vi "Timestamp I2C.vi"(0 "timestamp counter value":T2, 1 "reset":bool, 5 "i2c monitor array":T1[](array[typedef]) {"monitor word" format="%.0x"}) -> (4 "user timestamp fifo overflow":bool)   [LabVIEW 2020, in "GettingStarted_Common_148X_FPGA.lvlib"]
uses:
  GettingStarted_Common_148X_FPGA.lvlib
  <instrlib>/FlexRIO/CSI-2/v2/FPGA/Types/Timestamp Counter Value.ctl
  <instrlib>/FlexRIO/API/FPGA/v1/IO/NI148x/i2c monitor.ctl
  <instrlib>/_niInstr/Basic Elements/v1/FPGA/Private/Write U64 FIFO.vi
  <instrlib>/_niInstr/Basic Elements/v1/FPGA/niInstr Basic Elements v1 FPGA.lvlib
  <instrlib>/FlexRIO/CSI-2/v2/FPGA/NI CSI-2 API FPGA v2.lvlib
  <instrlib>/FlexRIO/CSI-2/v2/FPGA/subVIs/Convert User Timestamp to Raw Timestamp.vi
  <instrlib>/FlexRIO/CSI-2/v2/FPGA/Types/Timestamp ID.ctl
  <instrlib>/FlexRIO/API/FPGA/v1/IO/NI148x/FlexRIO 148x FPGA v1.lvlib
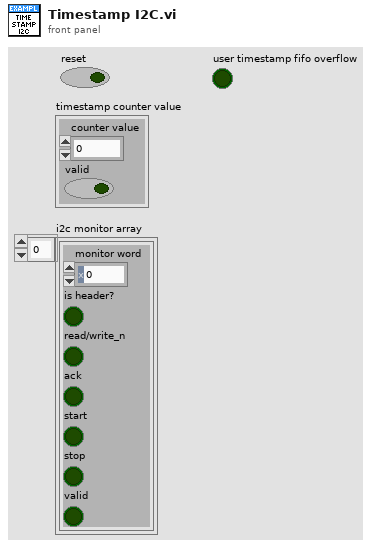
[diagram p1: front panel]
types:
  T1 = typedef "FlexRIO 148x FPGA v1.lvlib/i2c monitor.ctl" = cluster{"monitor word":u8, "is header?":bool, "read/write_n":bool, "ack":bool, "start":bool, "stop":bool, "valid":bool}
  T2 = typedef "NI CSI-2 API FPGA v2.lvlib/Timestamp Counter Value.ctl" = cluster{"counter value":u64, "valid":bool}
  T3 = typedef "NI CSI-2 API FPGA v2.lvlib/Timestamp ID.ctl" = enum8{"SI0 LLP", "SI1 LLP", "SI2 LLP", "SI3 LLP", "SI4 LLP", "SI5 LLP", "SI6 LLP", "SI7 LLP", "SO0 LLP", "SO1 LLP", "SO2 LLP", "SO3 LLP", "SO4 LLP", "SO5 LLP", "SO6 LLP", "SO7 LLP", "Ser0 GPIO Bank", "Ser1 GPIO Bank", "Ser2 GPIO Bank", "Ser3 GPIO Bank", "Ser4 GPIO Bank", "Ser5 GPIO Bank", "Ser6 GPIO Bank", "Ser7 GPIO Bank", "Des0 GPIO Bank", "Des1 GPIO Bank", "Des2 GPIO Bank", "Des3 GPIO Bank", "Des4 GPIO Bank", "Des5 GPIO Bank", "Des6 GPIO Bank", "Des7 GPIO Bank", "User0", "User1", "User2", "User3", "User4", "User5", "User6", "User7", "User8", "User9", "User10", "User11", "User12", "User13", "User14", "User15", "User16", "User17", "User18", "User19", "User20", "User21", "User22", "User23", "User24", "User25", "User26", "User27", "User28", "User29", "User30", "User31"}
  T4 = typedef "NI CSI-2 API FPGA v2.lvlib/User Timestamp.ctl" = cluster{"valid":bool, "user data":fxp<+,58,58>, "id":T3}
  T5 = typedef "NI CSI-2 API FPGA v2.lvlib/Raw Timestamp.ctl" = cluster{"timestamp":u64, "valid":bool}
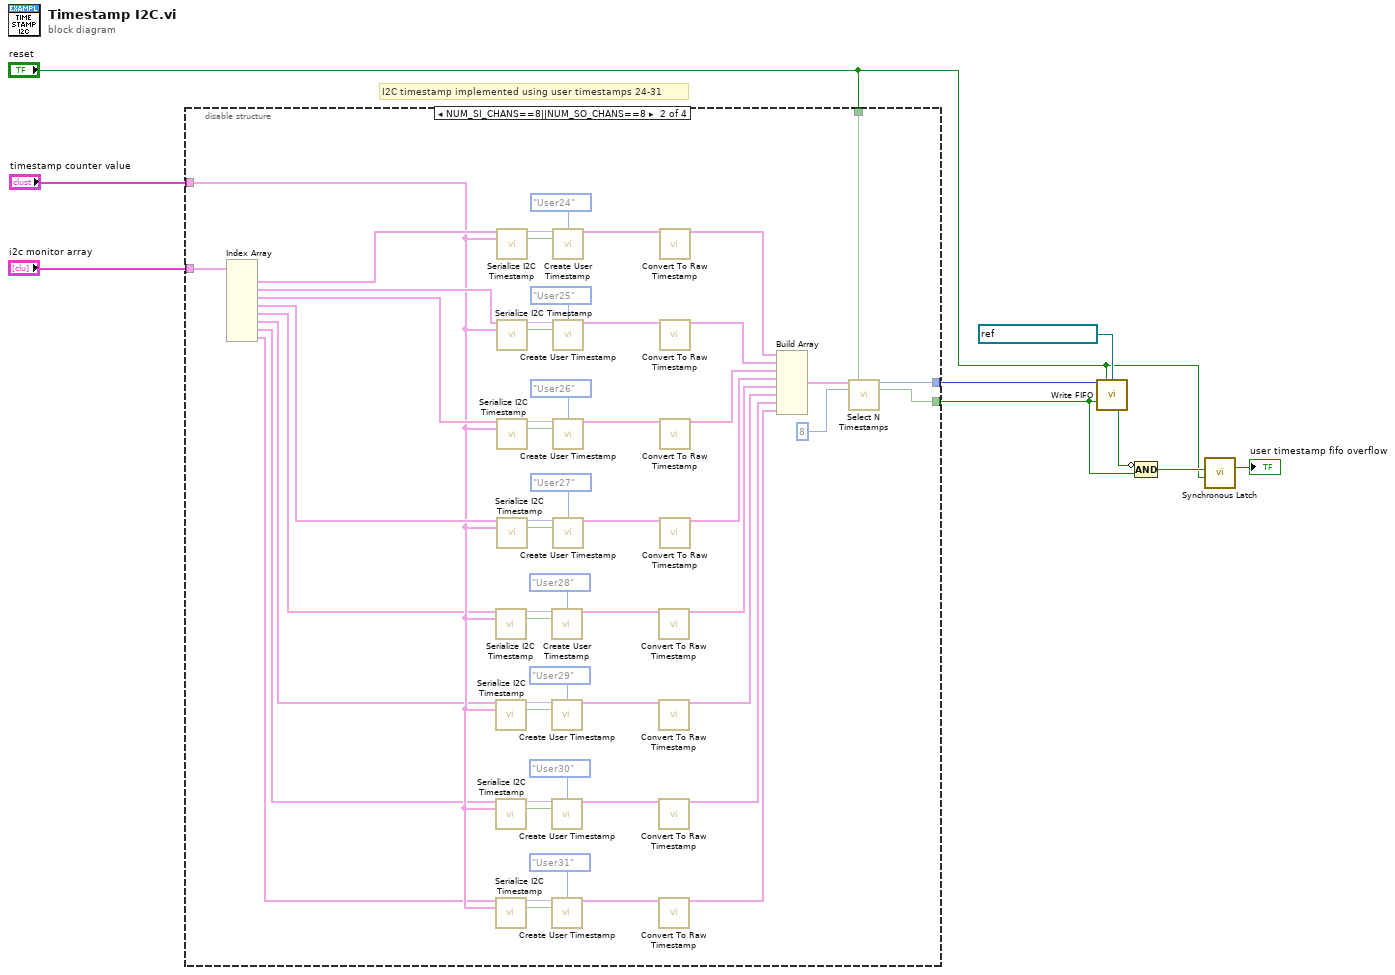
[diagram p0: block diagram]
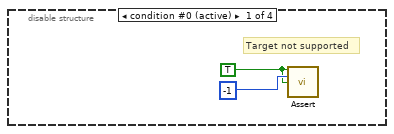
[diagram p2: hidden frame]
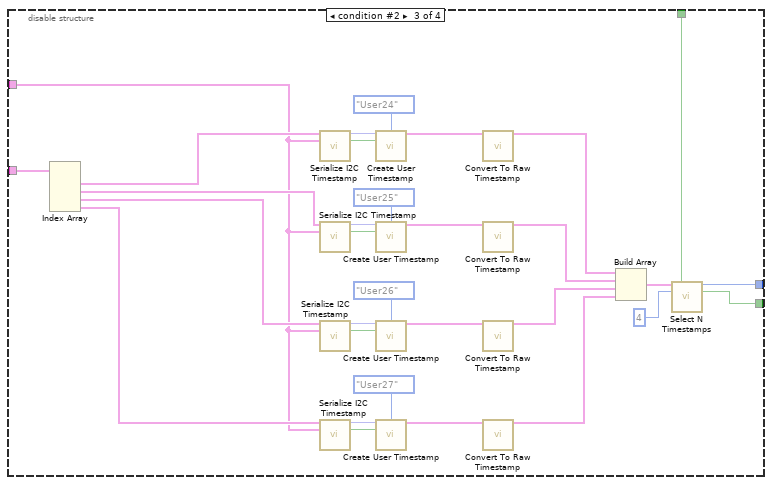
[diagram p3: hidden frame]
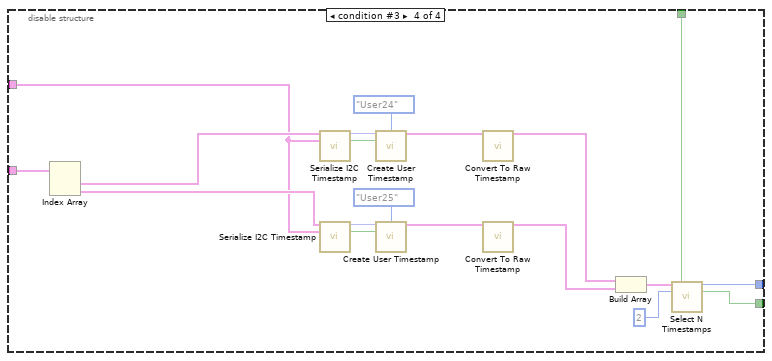
[diagram p4: hidden frame]
diagram:
  # "I2C timestamp implemented using user timestamps 24-31"
  n1 = disable-structure shown="NUM_SI_CHANS==8||NUM_SO_CHANS==8" {
    disable-tunnel: "i2c monitor array" -> [_ w42 w73 w104]
    disable-tunnel: "timestamp counter value" -> [_ w25 w72 w103]
    disable-tunnel: [_ w16 w70 w101] -> w3
    disable-tunnel: [_ w15 w69 w100] -> w2
    disable-tunnel: "reset" -> [_ w14 w68 w99]
    frame condition #0 (active) {
      w10 = TRUE ("assert")
      # "Target not supported"
      n2 = call <instrlib>:"Assert.vi"("assert"=w10, "error code"=-1, "enable show error"=w10) -> ()  [unwired: 13 in]
    }
    frame condition #1 {
      n3 = Index Array(array=w42) -> (element #1=w47:T1, element #2=w49:T1, element #3=w50:T1, element #4=w51:T1, element #5=w24:T1, element #6=w23:T1, element #7=w22:T1, element #8=w21:T1)  [unwired: 8 in]
      n4 = call "Serialize I2C Timestamp.vi"("i2c monitor"=w24, "timestamp counter value"=w25) -> ("data"=w39:fxp<+,58,58>, "create timestamp"=w38:bool)  [unwired: 12 in]
      n5 = call "Serialize I2C Timestamp.vi"("i2c monitor"=w23, "timestamp counter value"=w25) -> ("data"=w37:fxp<+,58,58>, "create timestamp"=w36:bool)  [unwired: 12 in]
      n6 = call "Serialize I2C Timestamp.vi"("i2c monitor"=w22, "timestamp counter value"=w25) -> ("data"=w35:fxp<+,58,58>, "create timestamp"=w34:bool)  [unwired: 12 in]
      n7 = call "Serialize I2C Timestamp.vi"("i2c monitor"=w21, "timestamp counter value"=w25) -> ("data"=w33:fxp<+,58,58>, "create timestamp"=w32:bool)  [unwired: 12 in]
      n8 = call "Serialize I2C Timestamp.vi"("i2c monitor"=w47, "timestamp counter value"=w25) -> ("data"=w45:fxp<+,58,58>, "create timestamp"=w46:bool)  [unwired: 12 in]
      n9 = call "Serialize I2C Timestamp.vi"("i2c monitor"=w49, "timestamp counter value"=w25) -> ("data"=w52:fxp<+,58,58>, "create timestamp"=w53:bool)  [unwired: 12 in]
      n10 = call "Serialize I2C Timestamp.vi"("i2c monitor"=w50, "timestamp counter value"=w25) -> ("data"=w54:fxp<+,58,58>, "create timestamp"=w55:bool)  [unwired: 12 in]
      n11 = call "Serialize I2C Timestamp.vi"("i2c monitor"=w51, "timestamp counter value"=w25) -> ("data"=w56:fxp<+,58,58>, "create timestamp"=w57:bool)  [unwired: 12 in]
      n12 = call <instrlib>:"Create User Timestamp.vi"("user data"=w39, "timestamp id"=Timestamp_ID."User28" ("id"), "create timestamp"=w38) -> ("user timestamp"=w41:T4)  [unwired: 12 in]
      n13 = call <instrlib>:"Create User Timestamp.vi"("user data"=w37, "timestamp id"=Timestamp_ID."User29" ("id"), "create timestamp"=w36) -> ("user timestamp"=w29:T4)  [unwired: 12 in]
      n14 = call <instrlib>:"Create User Timestamp.vi"("user data"=w35, "timestamp id"=Timestamp_ID."User30" ("id"), "create timestamp"=w34) -> ("user timestamp"=w30:T4)  [unwired: 12 in]
      n15 = call <instrlib>:"Create User Timestamp.vi"("user data"=w33, "timestamp id"=Timestamp_ID."User31" ("id"), "create timestamp"=w32) -> ("user timestamp"=w31:T4)  [unwired: 12 in]
      n16 = call <instrlib>:"Create User Timestamp.vi"("user data"=w45, "timestamp id"=Timestamp_ID."User24" ("id"), "create timestamp"=w46) -> ("user timestamp"=w43:T4)  [unwired: 12 in]
      n17 = call <instrlib>:"Create User Timestamp.vi"("user data"=w52, "timestamp id"=Timestamp_ID."User25" ("id"), "create timestamp"=w53) -> ("user timestamp"=w60:T4)  [unwired: 12 in]
      n18 = call <instrlib>:"Create User Timestamp.vi"("user data"=w54, "timestamp id"=Timestamp_ID."User26" ("id"), "create timestamp"=w55) -> ("user timestamp"=w59:T4)  [unwired: 12 in]
      n19 = call <instrlib>:"Create User Timestamp.vi"("user data"=w56, "timestamp id"=Timestamp_ID."User27" ("id"), "create timestamp"=w57) -> ("user timestamp"=w58:T4)  [unwired: 12 in]
      n20 = call-poly <instrlib>:"Convert To Raw Timestamp.vi"("user timestamp"=w41) -> ("raw timestamp"=w20:T5)  [unwired: 14 in]
      n21 = call-poly <instrlib>:"Convert To Raw Timestamp.vi"("user timestamp"=w29) -> ("raw timestamp"=w19:T5)  [unwired: 14 in]
      n22 = call-poly <instrlib>:"Convert To Raw Timestamp.vi"("user timestamp"=w30) -> ("raw timestamp"=w18:T5)  [unwired: 14 in]
      n23 = call-poly <instrlib>:"Convert To Raw Timestamp.vi"("user timestamp"=w31) -> ("raw timestamp"=w17:T5)  [unwired: 14 in]
      n24 = call-poly <instrlib>:"Convert To Raw Timestamp.vi"("user timestamp"=w43) -> ("raw timestamp"=w48:T5)  [unwired: 14 in]
      n25 = call-poly <instrlib>:"Convert To Raw Timestamp.vi"("user timestamp"=w60) -> ("raw timestamp"=w61:T5)  [unwired: 14 in]
      n26 = call-poly <instrlib>:"Convert To Raw Timestamp.vi"("user timestamp"=w59) -> ("raw timestamp"=w62:T5)  [unwired: 14 in]
      n27 = call-poly <instrlib>:"Convert To Raw Timestamp.vi"("user timestamp"=w58) -> ("raw timestamp"=w63:T5)  [unwired: 14 in]
      n28 = Build Array(w48, w61, w62, w63, w20, w19, w18, w17) -> (w13:T5[])
      n29 = call <instrlib>:"Select N Timestamps.vi"("raw timestamps"=w13, "reset"=w14, "number of timestamps"=u8 8) -> ("timestamp"=w16:u64, "output valid"=w15:bool)  [unwired: 11 in]
    }
    frame condition #2 {
      n30 = Index Array(array=w73) -> (element #1=w78:T1, element #2=w80:T1, element #3=w81:T1, element #4=w82:T1)  [unwired: 4 in]
      n31 = call "Serialize I2C Timestamp.vi"("i2c monitor"=w78, "timestamp counter value"=w72) -> ("data"=w76:fxp<+,58,58>, "create timestamp"=w77:bool)  [unwired: 12 in]
      n32 = call "Serialize I2C Timestamp.vi"("i2c monitor"=w80, "timestamp counter value"=w72) -> ("data"=w83:fxp<+,58,58>, "create timestamp"=w84:bool)  [unwired: 12 in]
      n33 = call "Serialize I2C Timestamp.vi"("i2c monitor"=w81, "timestamp counter value"=w72) -> ("data"=w85:fxp<+,58,58>, "create timestamp"=w86:bool)  [unwired: 12 in]
      n34 = call "Serialize I2C Timestamp.vi"("i2c monitor"=w82, "timestamp counter value"=w72) -> ("data"=w87:fxp<+,58,58>, "create timestamp"=w88:bool)  [unwired: 12 in]
      n35 = call <instrlib>:"Create User Timestamp.vi"("user data"=w76, "timestamp id"=Timestamp_ID."User24" ("id"), "create timestamp"=w77) -> ("user timestamp"=w74:T4)  [unwired: 12 in]
      n36 = call <instrlib>:"Create User Timestamp.vi"("user data"=w83, "timestamp id"=Timestamp_ID."User25" ("id"), "create timestamp"=w84) -> ("user timestamp"=w91:T4)  [unwired: 12 in]
      n37 = call <instrlib>:"Create User Timestamp.vi"("user data"=w85, "timestamp id"=Timestamp_ID."User26" ("id"), "create timestamp"=w86) -> ("user timestamp"=w90:T4)  [unwired: 12 in]
      n38 = call <instrlib>:"Create User Timestamp.vi"("user data"=w87, "timestamp id"=Timestamp_ID."User27" ("id"), "create timestamp"=w88) -> ("user timestamp"=w89:T4)  [unwired: 12 in]
      n39 = call-poly <instrlib>:"Convert To Raw Timestamp.vi"("user timestamp"=w74) -> ("raw timestamp"=w79:T5)  [unwired: 14 in]
      n40 = call-poly <instrlib>:"Convert To Raw Timestamp.vi"("user timestamp"=w91) -> ("raw timestamp"=w92:T5)  [unwired: 14 in]
      n41 = call-poly <instrlib>:"Convert To Raw Timestamp.vi"("user timestamp"=w90) -> ("raw timestamp"=w93:T5)  [unwired: 14 in]
      n42 = call-poly <instrlib>:"Convert To Raw Timestamp.vi"("user timestamp"=w89) -> ("raw timestamp"=w94:T5)  [unwired: 14 in]
      n43 = Build Array(w79, w92, w93, w94) -> (w71:T5[])
      n44 = call <instrlib>:"Select N Timestamps.vi"("raw timestamps"=w71, "reset"=w68, "number of timestamps"=u8 4) -> ("timestamp"=w70:u64, "output valid"=w69:bool)  [unwired: 11 in]
    }
    frame condition #3 {
      n45 = Index Array(array=w104) -> (element #1=w109:T1, element #2=w111:T1)  [unwired: 2 in]
      n46 = call "Serialize I2C Timestamp.vi"("i2c monitor"=w109, "timestamp counter value"=w103) -> ("data"=w107:fxp<+,58,58>, "create timestamp"=w108:bool)  [unwired: 12 in]
      n47 = call "Serialize I2C Timestamp.vi"("i2c monitor"=w111, "timestamp counter value"=w103) -> ("data"=w112:fxp<+,58,58>, "create timestamp"=w113:bool)  [unwired: 12 in]
      n48 = call <instrlib>:"Create User Timestamp.vi"("user data"=w107, "timestamp id"=Timestamp_ID."User24" ("id"), "create timestamp"=w108) -> ("user timestamp"=w105:T4)  [unwired: 12 in]
      n49 = call <instrlib>:"Create User Timestamp.vi"("user data"=w112, "timestamp id"=Timestamp_ID."User25" ("id"), "create timestamp"=w113) -> ("user timestamp"=w114:T4)  [unwired: 12 in]
      n50 = call-poly <instrlib>:"Convert To Raw Timestamp.vi"("user timestamp"=w105) -> ("raw timestamp"=w110:T5)  [unwired: 14 in]
      n51 = call-poly <instrlib>:"Convert To Raw Timestamp.vi"("user timestamp"=w114) -> ("raw timestamp"=w115:T5)  [unwired: 14 in]
      n52 = Build Array(w110, w115) -> (w102:T5[])
      n53 = call <instrlib>:"Select N Timestamps.vi"("raw timestamps"=w102, "reset"=w99, "number of timestamps"=u8 2) -> ("timestamp"=w101:u64, "output valid"=w100:bool)  [unwired: 11 in]
    }
  }
  n54 = call-poly <instrlib>:"Write FIFO.vi"("input data"=w3, "reset"="reset", "fifo"=refnum<k21> "User Timestamps" ("FIFO In"), "input valid"=w2) -> ("ready for input"=w8:bool)  [unwired: 11 in]
  n55 = Compound Arithmetic op=AND(invert w8, w2) -> (w4:bool)
  n56 = call <instrlib>:"Synchronous Latch.vi"("clear"="reset", "set"=w4) -> ("out"=→"user timestamp fifo overflow":bool)  [unwired: 9 in]
